vi "Write test data to sql.vi"(8 "error in (no error)":errorcluster) -> (0 "error out":errorcluster)   [LabVIEW 2013]
uses:
  Main Support/Global 2.vi
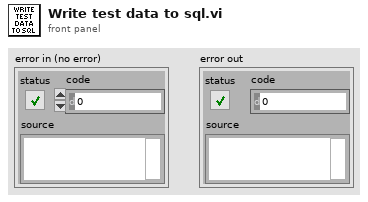
[diagram p1: front panel]
types:
  T1 = enum16{"Query", "Insert", "Select", "Dump Recs", "Get Rec Count", "Get Col Names", "Insert all fields", "Find", "Get last test result"}
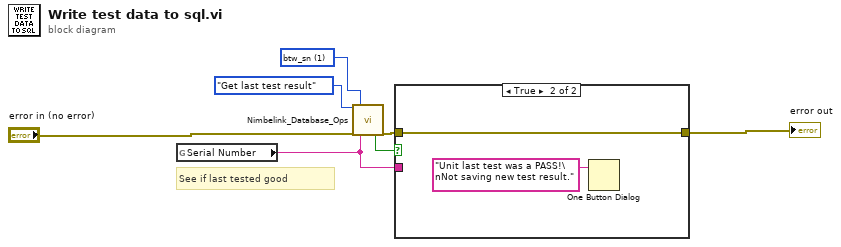
[diagram p0: block diagram]
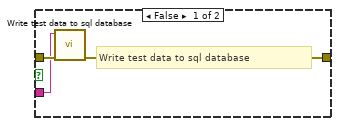
[diagram p2: hidden frame]
diagram:
  w3 = u16 1 items=["work_order", "btw_sn", "mac", "meid", "operator", "datetime", "part_number", "imei", "sim_id", "phone", "test_result"] ("Find column")
  # "See if last tested good"
  n1 = global read "Global 2.vi" "Serial Number"() -> (w1:string)
  n2 = call "Nimbelink_Database_Ops.vi"("Operation"=T1."Get last test result", "Error in (no error)"="error in (no error)", "Find column"=w3, "Find data"=w1) -> ("Last test passed?"=w5:bool, "Error out"=w2:errorcluster)  [unwired: 8 in, 6 out]
  n3 = case shown="True" w5 {
    tunnel: w2 -> [w10 w12]
    tunnel: [w9 w12] -> w7
    tunnel: w1 -> [w8 _]
    frame False {
      # "Write test data to sql database"
      n4 = call "Write test data to sql database.vi"("error in (no error)"=w10, "Serial"=w8) -> ("error out"=w9:errorcluster)  [unwired: 4 in, 3 out]
    }
    frame True {
      n5 = One Button Dialog(message="Unit last test was a PASS!\nNot saving new test result.") -> ()  [unwired: 1 in, 1 out]
    }
  }
  "error out" <- w7
